vi "Data.Numeric Limits to String Items.vi"(8 "UL":dbl, 9 "LL":dbl, 10 "LimType":T1, 11 "Value":dbl) -> (0 "UL":string, 1 "LL":string, 2 "LimType":string, 3 "Value":string)   [LabVIEW 2024, in "EQMF.lvlib" / "Data.lvlib"]
uses:
  Data.lvlib
  TypeDefs/Data.Result Numeric Limit Type.ctl
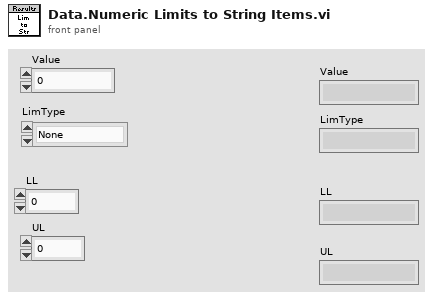
[diagram p1: front panel]
types:
  T1 = typedef "EQMF.lvlib/Data.lvlib/Data.Result Numeric Limit Type.ctl" = enum16{"None", "EQ", "NE", "GT", "LT", "GE", "LE", "GTLT", "GELE", "GELT", "GTLE", "LTGT", "LEGE", "LEGT", "LTGE"}
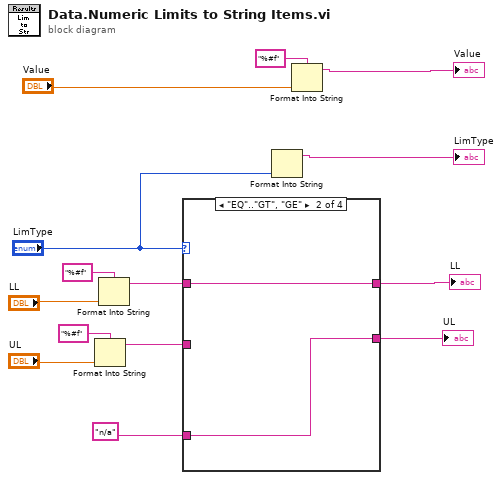
[diagram p0: block diagram]
diagram:
  n1 = Format Into String(format string="%#f", "UL") -> (resulting string=w9:string)  [unwired: 2 in, 1 out]
  n2 = Format Into String(format string="%#f", "LL") -> (resulting string=w10:string)  [unwired: 2 in, 1 out]
  n3 = case shown="\"EQ\"..\"GT\", \"GE\"" "LimType" {
    tunnel: w10 -> [_ w17 _ w20]
    tunnel: w9 -> [_ _ w18 w21]
    tunnel: "n/a" ("N/A Filler") -> [w15 w16 w19 _]
    tunnel: [w15 w17 w19 w20] -> w5
    tunnel: [w15 w16 w18 w21] -> w4
    frame "None" {
    }
    frame "EQ".."GT", "GE" {
    }
    frame "LT", "LE" {
    }
    frame Default {
    }
  }
  "LL" <- w5
  "UL" <- w4
  n4 = Format Into String("LimType") -> (resulting string=→"LimType":string)  [unwired: 3 in, 1 out]
  n5 = Format Into String(format string="%#f", "Value") -> (resulting string=→"Value":string)  [unwired: 2 in, 1 out]
